vi "add type to string.vi"(10 "Interface Type":T1, 11 "Alias":string) -> (3 "Alias with Type Appended":string)   [LabVIEW 2015]
uses:
  Shared/Controls/Interface Type.ctl
  Shared/Modbus Master Shared.lvlib
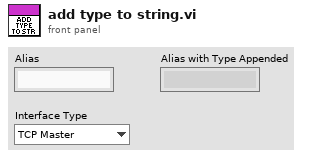
[diagram p1: front panel]
types:
  T1 = typedef "Modbus Master Shared.lvlib/Interface Type.ctl" = enum16{"TCP Master", "Serial Master"}
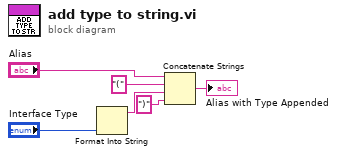
[diagram p0: block diagram]
diagram:
  n1 = Format Into String("Interface Type") -> (resulting string=w3:string)  [unwired: 3 in, 1 out]
  n2 = Concatenate Strings("Alias", "(" ("string"), w3, ")" ("string")) -> (→"Alias with Type Appended":string)
